vi "PageSelectorValueChange.vi"(8 "error in (no error)":errorcluster, 10 "NewVal":i32, 11 "View in":refnum<class "View.lvclass">) -> (0 "error out":errorcluster, 3 "View out":refnum<class "View.lvclass">)   [LabVIEW 2020, in "Container.lvlib" / "View.lvclass"]
uses:
  View.lvclass
  View.lvclass/View.ctl
  Controller/Controller.lvclass
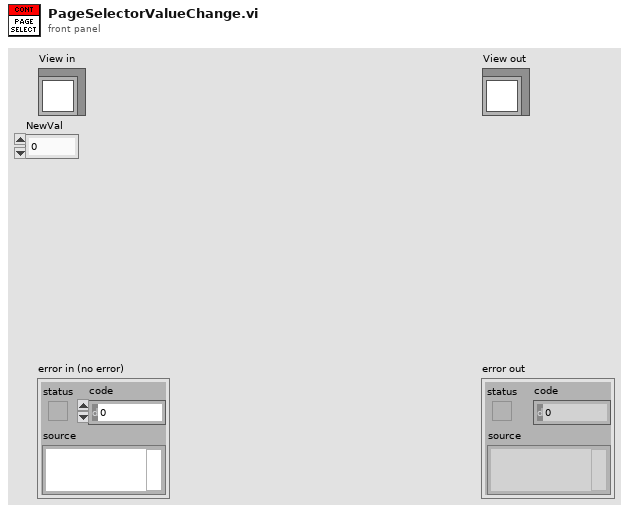
[diagram p1: front panel]
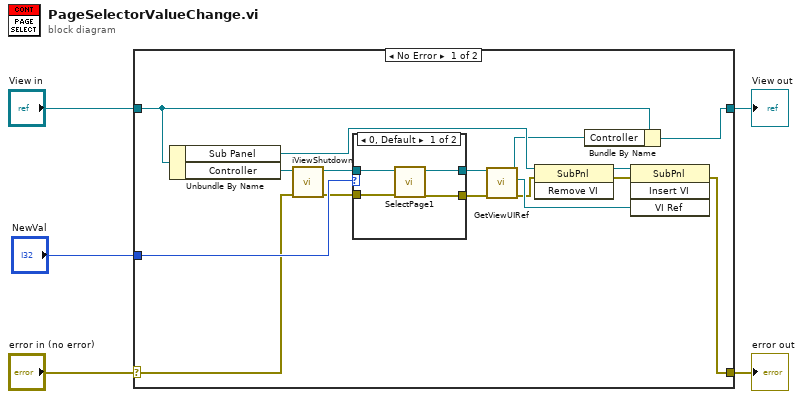
[diagram p0: block diagram]
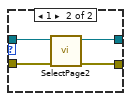
[diagram p2: hidden frame]
diagram:
  n1 = case shown="No Error" "error in (no error)" {
    selector: "error in (no error)" -> [w10 w31]
    tunnel: [w9 w31] -> w4
    tunnel: [w6 w30] -> w2
    tunnel: "View in" -> [w8 w30]
    tunnel: "NewVal" -> [w20 _]
    frame No Error {
      n2 = Unbundle By Name(w8) -> ("Sub Panel"=w15:refnum<vi>, "Controller"=w21:refnum<class "Controller.lvclass">)
      n3 = call "iViewShutdown.vi"("error in (no error)"=w10, "Controller in"=w21) -> ("error out"=w11:errorcluster, "Controller out"=w19:refnum<class "Controller.lvclass">)  [unwired: 8 in]
      n4 = case shown="0, Default" w20 {
        tunnel: w19 -> [w25 w29]
        tunnel: [w24 w28] -> w18
        tunnel: [w23 w27] -> w12
        tunnel: w11 -> [w22 w26]
        frame 0, Default {
          n5 = call "SelectPage1.vi"("error in (no error)"=w22, "Controller in"=w25) -> ("error out"=w23:errorcluster, "Controller out"=w24:refnum<class "Controller.lvclass">)  [unwired: 8 in]
        }
        frame 1 {
          n6 = call "SelectPage2.vi"("error in (no error)"=w26, "Controller in"=w29) -> ("error out"=w27:errorcluster, "Controller out"=w28:refnum<class "Controller.lvclass">)  [unwired: 8 in]
        }
      }
      n7 = call "GetViewUIRef.vi"("error in (no error)"=w12, "Controller in"=w18) -> ("error out"=w13:errorcluster, "UIRef"=w17:refnum<vi>, "Controller out"=w7:refnum<class "Controller.lvclass">)  [unwired: 7 in]
      n8 = invoke class="SubPnl" method="Remove VI"(reference=w15, error in=w13) -> (reference out=w14:refnum<vi>, error out=w16:errorcluster)  [unwired: 1 in, 1 out]
      n9 = Bundle By Name(cluster=w8, "Controller"=w7) -> (w6:refnum<class "View.lvclass">)
      n10 = invoke class="SubPnl" method="Insert VI"(reference=w14, error in=w16, "VI Ref"=w17) -> (error out=w9:errorcluster)  [unwired: 1 in, 3 out]
    }
    frame Error {
    }
  }
  "error out" <- w4
  "View out" <- w2
